vi "Autonomous Independent.vi"   [LabVIEW 2012]
doc: "This VI is called when autonomous begins, and will automatically be terminated when autonomous ends. You can carry out timed or sensor driven robot movement independently without needing to return to the caller."
uses:
  Robot Global Data.vi
  <vilib>/Rock Robotics/WPI/Joystick/WPI_JoystickGetSetRefNum.vi
panel:
  # "Be sure to right-click and choose Data Operations>>Make Current Value default if you want to save the array values with the VI"
types:
  T1 = typedef "WPI_JoystickDevRef.ctl" = cluster{"Device":T2}
  T2 = typedef "WPI_JoystickDeviceEnum.ctl" = enum16{"USB 1", "USB 2", "USB 3", "USB 4", "Kinect 1", "Kinect 2"}
  T3 = cluster{"axis 1 (x)":dbl, "axis 2 (y)":dbl, "axis 3 (throttle)":dbl, "axis 4":dbl, "axis 5":dbl, "axis 6":dbl}
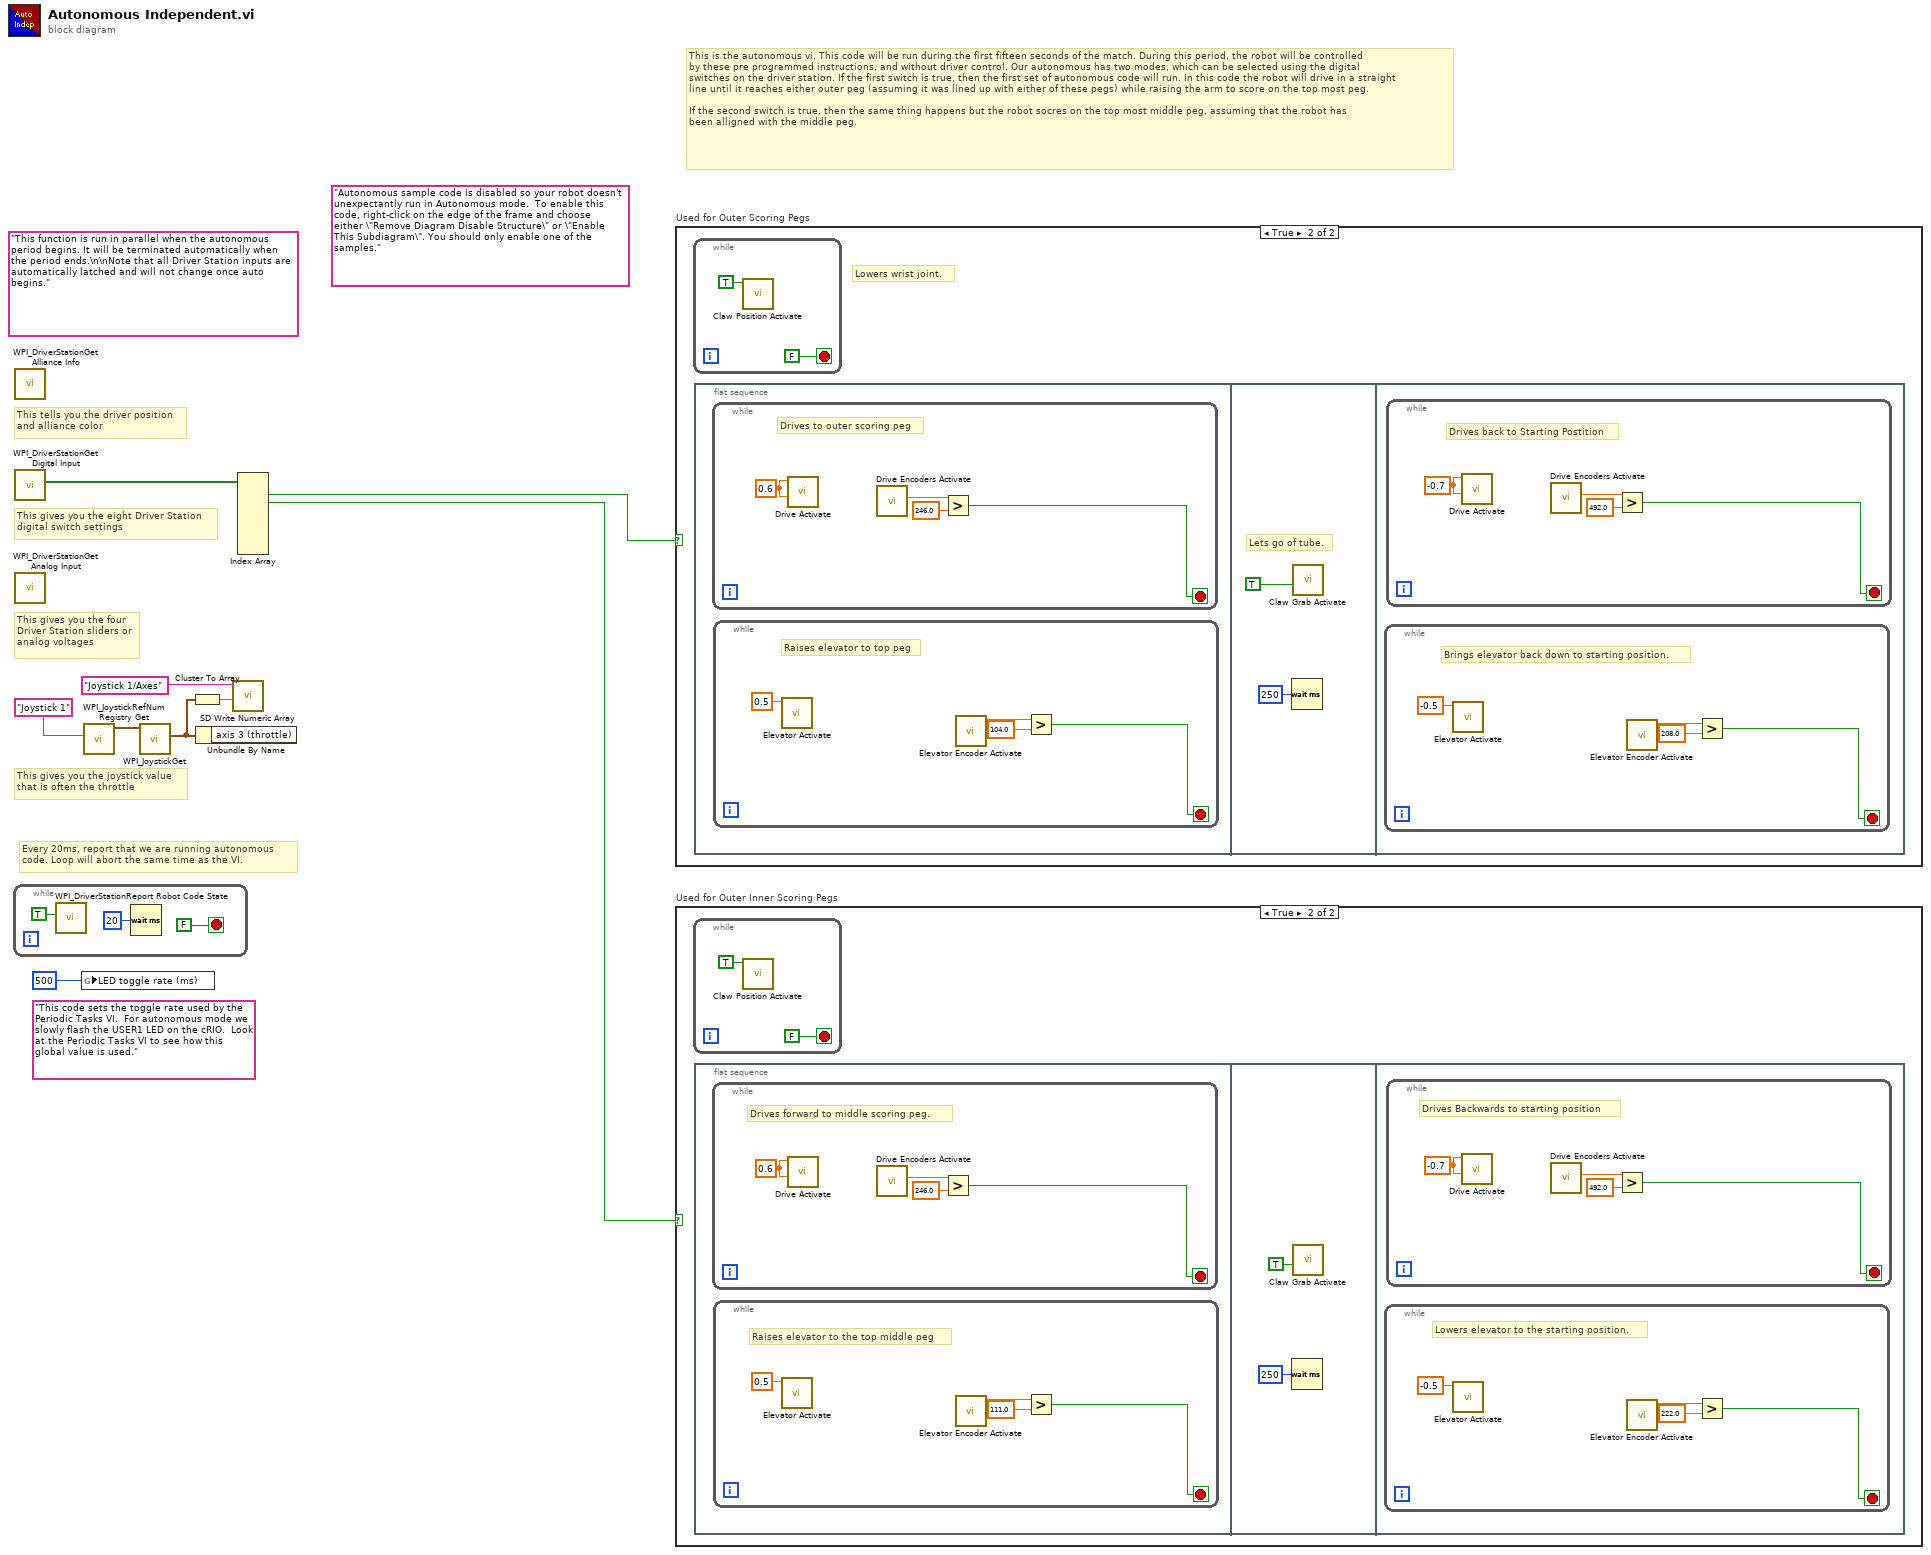
[diagram p0: block diagram]
diagram:
  (unwired) "This code sets the toggle rate used by the Periodic Tasks VI.  For autonomous mode we slowly flash the USER1 LED on the cRIO.  Look at the Periodic Tasks VI to see how this global value is used."
  (unwired) "Autonomous sample code is disabled so your robot doesn't unexpectantly run in Autonomous mode.  To enable this code, right-click on the edge of the frame and choose either \"Remove Diagram Disable Structure\" or \"Enable This Subdiagram\". You should only enable one of the samples."
  (unwired) "This function is run in parallel when the autonomous period begins. It will be terminated automatically when the period ends.\n\nNote that all Driver Station inputs are automatically latched and will not change once auto begins."
  # "This is the autonomous vi. This code will be run during the first fifteen seconds of the match. During this period, the robot will be controlled \nby these pre programmed instructions, and without driver control. Our autonomous has two modes, which can be selected using the digital \nswitches on the driver station. If the first switch is true, then the first set of autonomous code will run. In this code the robot will drive in a straight\nline until it reaches either outer peg (assuming it was lined up with either of these pegs) while raising the arm to score on the top most peg. \n\nIf the second switch is true, then the same thing happens but the robot socres on the top most middle peg, assuming that the robot has \nbeen alligned with the middle peg."
  # "Every 20ms, report that we are running autonomous\ncode. Loop will abort the same time as the VI."
  # "This gives you the joystick value\nthat is often the throttle"
  # "This tells you the driver position\nand alliance color"
  # "This gives you the eight Driver Station\ndigital switch settings"
  # "This gives you the four\nDriver Station sliders or\nanalog voltages"
  n1 = while {
    stop <- FALSE stop-if-true
    n2 = call <vilib>:"WPI_DriverStationReport Robot Code State.vi"("Autonomous"=TRUE) -> ()  [unwired: 10 in, 1 out]
    n3 = Wait (ms)(milliseconds to wait=u32 20) -> ()  [unwired: 1 out]
  }
  n4 = call <vilib>:"WPI_DriverStationGet Alliance Info.vi"() -> ()  [unwired: 12 out]
  n5 = call <vilib>:"WPI_DriverStationGet Digital Input.vi"() -> ("Driver Station Digital Input (1-8)"=w9:bool[])  [unwired: 11 out]
  n6 = call <vilib>:"WPI_DriverStationGet Analog Input.vi"() -> ()  [unwired: 12 out]
  n7 = global write "Robot Global Data.vi" "LED toggle rate (ms)"(u32 500 ("LED ms toggle rate")) -> ()
  n8 = call <vilib>:"WPI_JoystickRefNum Registry Get.vi"("refnum name"="Joystick 1") -> ("JoystickDevRef"=w7:T1)  [unwired: 1 in, 9 out]
  n9 = call <vilib>:"WPI_JoystickGet.vi"("JoystickDevRef"=w7) -> ("Axes"=w4:T3)  [unwired: 1 in, 5 out]
  n10 = Cluster To Array(cluster=w4) -> (array=w5:dbl[])
  n11 = Unbundle By Name(w4) -> ()  [unwired: 1 out]
  n12 = call <vilib>:"SD Write Numeric Array.vi"("Numeric Array"=w5, "Name"="Joystick 1/Axes") -> ()  [unwired: 8 in, 2 out]
  n13 = Index Array(array=w9) -> (element #1=w2:bool, element #2=w1:bool)  [unwired: 8 in, 6 out]
  n14 = case "Used for Outer Scoring Pegs" shown="True" w2 {
    frame False {
    }
    frame True {
      # "Lowers wrist joint."
      n15 = while {
        stop <- FALSE stop-if-true
        n16 = call "Claw Position Activate.vi"("Claw Extend"=TRUE) -> ()  [unwired: 11 in]
      }
      n17 = flat-sequence {
        frame #0 {
          n18 = while {
            stop <- w19 stop-if-true
            w22 = 0.6 ("Left Joystick")
            # "Drives to outer scoring peg"
            n19 = call "Drive Activate.vi"("Right Joystick"=w22, "Left Joystick"=w22) -> ()  [unwired: 10 in]
            n20 = call "Drive Encoders Activate.vi"() -> ("Distance"=w21:dbl)  [unwired: 11 in]
            n21 = Greater?(x=w21, y=246.0) -> (0:w19:bool)
          }
          n22 = while {
            stop <- w15 stop-if-true
            # "Raises elevator to top peg"
            n23 = call "Elevator Activate.vi"("Elevator Output"=0.5) -> ()  [unwired: 11 in]
            n24 = call "Elevator Encoder Activate.vi"() -> ("Distance"=w17:dbl)  [unwired: 11 in]
            n25 = Greater?(x=w17, y=104.0) -> (0:w15:bool)
          }
        }
        frame #1 {
          # "Lets go of tube."
          n26 = Wait (ms)(milliseconds to wait=u32 250) -> ()  [unwired: 1 out]
          n27 = call "Claw Grab Activate.vi"("Let Go"=TRUE) -> ()  [unwired: 11 in]
        }
        frame #2 {
          n28 = while {
            stop <- w25 stop-if-true
            # "Brings elevator back down to starting position."
            n29 = call "Elevator Activate.vi"("Elevator Output"=-0.5) -> ()  [unwired: 11 in]
            n30 = call "Elevator Encoder Activate.vi"() -> ("Distance"=w27:dbl)  [unwired: 11 in]
            n31 = Greater?(x=w27, y=208.0) -> (0:w25:bool)
          }
          n32 = while {
            stop <- w29 stop-if-true
            w32 = -0.7 ("Left Joystick")
            # "Drives back to Starting Postition"
            n33 = call "Drive Activate.vi"("Right Joystick"=w32, "Left Joystick"=w32) -> ()  [unwired: 10 in]
            n34 = call "Drive Encoders Activate.vi"() -> ("Distance"=w31:dbl)  [unwired: 11 in]
            n35 = Greater?(x=w31, y=492.0) -> (0:w29:bool)
          }
        }
      }
    }
  }
  n36 = case "Used for Outer Inner Scoring Pegs" shown="True" w1 {
    frame False {
    }
    frame True {
      n37 = while {
        stop <- FALSE stop-if-true
        n38 = call "Claw Position Activate.vi"("Claw Extend"=TRUE) -> ()  [unwired: 11 in]
      }
      n39 = flat-sequence {
        frame #0 {
          n40 = while {
            stop <- w39 stop-if-true
            w42 = 0.6 ("Left Joystick")
            # "Drives forward to middle scoring peg."
            n41 = call "Drive Activate.vi"("Right Joystick"=w42, "Left Joystick"=w42) -> ()  [unwired: 10 in]
            n42 = call "Drive Encoders Activate.vi"() -> ("Distance"=w41:dbl)  [unwired: 11 in]
            n43 = Greater?(x=w41, y=246.0) -> (0:w39:bool)
          }
          n44 = while {
            stop <- w35 stop-if-true
            # "Raises elevator to the top middle peg"
            n45 = call "Elevator Activate.vi"("Elevator Output"=0.5) -> ()  [unwired: 11 in]
            n46 = call "Elevator Encoder Activate.vi"() -> ("Distance"=w37:dbl)  [unwired: 11 in]
            n47 = Greater?(x=w37, y=111.0) -> (0:w35:bool)
          }
        }
        frame #1 {
          n48 = Wait (ms)(milliseconds to wait=u32 250) -> ()  [unwired: 1 out]
          n49 = call "Claw Grab Activate.vi"("Let Go"=TRUE) -> ()  [unwired: 11 in]
        }
        frame #2 {
          n50 = while {
            stop <- w45 stop-if-true
            # "Lowers elevator to the starting position."
            n51 = call "Elevator Activate.vi"("Elevator Output"=-0.5) -> ()  [unwired: 11 in]
            n52 = call "Elevator Encoder Activate.vi"() -> ("Distance"=w47:dbl)  [unwired: 11 in]
            n53 = Greater?(x=w47, y=222.0) -> (0:w45:bool)
          }
          n54 = while {
            stop <- w49 stop-if-true
            w52 = -0.7 ("Left Joystick")
            # "Drives Backwards to starting position"
            n55 = call "Drive Activate.vi"("Right Joystick"=w52, "Left Joystick"=w52) -> ()  [unwired: 10 in]
            n56 = call "Drive Encoders Activate.vi"() -> ("Distance"=w51:dbl)  [unwired: 11 in]
            n57 = Greater?(x=w51, y=492.0) -> (0:w49:bool)
          }
        }
      }
    }
  }
